vi "ep_Decimate Harmonics.vi"(10 "decimation factor":i32, 11 "array in":cdb[](array[numeric])) -> (3 "decimated array":cdb[](array[numeric]))   [LabVIEW 2013, in "NI_EP_Power Measurement.lvlib"]
uses:
  <vilib>/addons/Electrical Power/Power Measurement/NI_EP_Power Measurement.lvlib
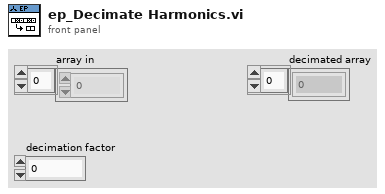
[diagram p1: front panel]
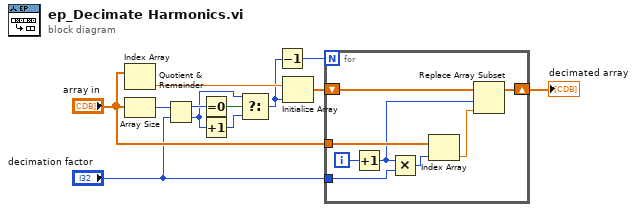
[diagram p0: block diagram]
diagram:
  n1 = Index Array(array="array in") -> (element=w7:cdb)  [unwired: 1 in]
  n2 = Array Size(array="array in") -> (size(s)=w12:i32)
  n3 = Quotient & Remainder(x=w12, y="decimation factor") -> (x-y*floor(x/y)=w11:i32, floor(x/y)=w8:i32)
  n4 = Equal To 0?(x=w11) -> (x = 0?=w10:bool)
  n5 = Increment(x=w8) -> (x+1=w9:i32)
  n6 = Select(t=w8, s=w10, f=w9) -> (s? t:f=w5:i32)
  n7 = Decrement(x=w5) -> (x-1=w6:i32)
  n8 = Initialize Array(w7, w5) -> (w4:cdb[])
  n9 = for {
    N: w6 -> [_]
    shift-right: [w16] -> w3
    shift-left: w4 -> [w17]
    tunnel: "array in" -> [w20]
    tunnel: "decimation factor" -> [w13]
    i -> [w19]
    n10 = Increment(x=w19) -> (x+1=w14:i32)
    n11 = Multiply(x=w14, y=w13) -> (x*y=w18:i32)
    n12 = Index Array(array=w20, index=w18) -> (element=w15:cdb)
    n13 = Replace Array Subset(array=w17, new element=w15, index=w14) -> (w16:cdb[])
  }
  "decimated array" <- w3
